vi "num2bool.vi"(11 "INTERGER ARRAY":i64[](array[numeric])) -> (3 "BOOLEAN ARRAY":bool[](array[boolean]))   [LabVIEW 2013]
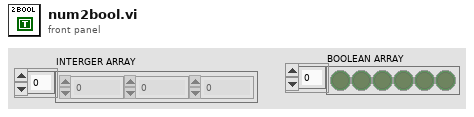
[diagram p1: front panel]
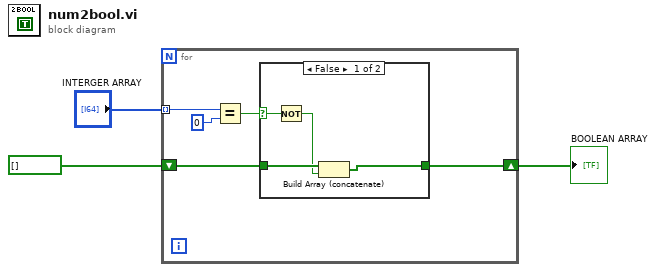
[diagram p0: block diagram]
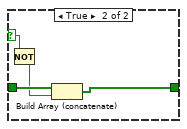
[diagram p2: hidden frame]
diagram:
  n1 = for {
    tunnel: "INTERGER ARRAY" -> [w8] mode=indexing
    shift-right: [w4] -> w1
    shift-left: bool[] [] -> [w5]
    n2 = Equal?(x=w8, y=i64 0) -> (x = y?=w6:bool)
    n3 = case shown="False" w6 {
      selector: w6 -> [w10 w15]
      tunnel: w5 -> [w12 w16]
      tunnel: [w11 w13] -> w4
      frame False {
        n4 = Not(x=w10) -> (.not. x?=w9:bool)
        n5 = Build Array (concatenate)(w12, w9) -> (w11:bool[])
      }
      frame True {
        n6 = Not(x=w15) -> (.not. x?=w14:bool)
        n7 = Build Array (concatenate)(w16, w14) -> (w13:bool[])
      }
    }
  }
  "BOOLEAN ARRAY" <- w1
